vi "3D Major Grid.vi"(5 "Grid Plane Visible":T1, 6 "Inverted?":bool, 7 "Axis":enum16{"X-Axis", "Y-Axis", "Z-Axis"}(ring), 8 "error in (no error)":errorcluster, 9 "Grid Color":u32(colorbox), 10 "Range":cluster{"Max":sgl, "Min":sgl}, 11 "Tick Cluster Array":T2) -> (0 "error out":errorcluster, 3 "Grid Object Out":refnum<vi>)   [LabVIEW 2013]
uses:
  <vilib>/Math Plots/3D Math Plots/3D Plot/3D Plot/Typedef/Tick Array.ctl
  <vilib>/picture/3D Picture Control/Object/Create Object (name).vi
  <vilib>/picture/3D Picture Control/NI_3D Picture Control.lvlib
  <vilib>/Math Plots/3D Math Plots/3D Plot/3D Plot/3D Plot.lvclass
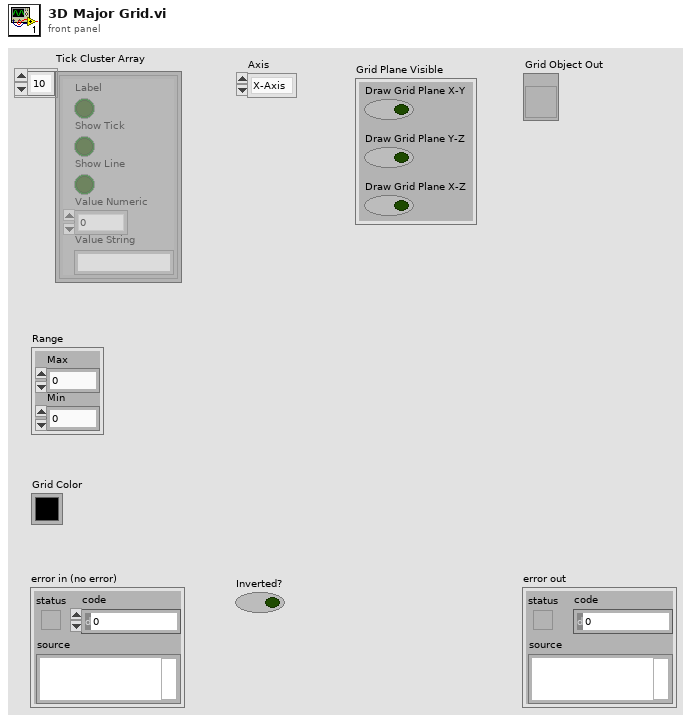
[diagram p1: front panel]
types:
  T1 = cluster{"Draw Grid Plane X-Y":bool, "Draw Grid Plane Y-Z":bool, "Draw Grid Plane X-Z":bool}
  T2 = typedef "3D Plot.lvclass/Tick Array.ctl" = cluster{"Label":bool, "Show Tick":bool, "Show Line":bool, "Value Numeric":sgl, "Value String":string}[]
  T3 = enum16{"Overall", "Per Primitive", "Per Vertex", "Binding Off"}
  T4 = enum16{"Points", "Lines", "Line Strip", "Line Loop", "Triangles", "Triangle Strip", "Triangle Fan", "Quads", "Quad Strip", "Polygon"}
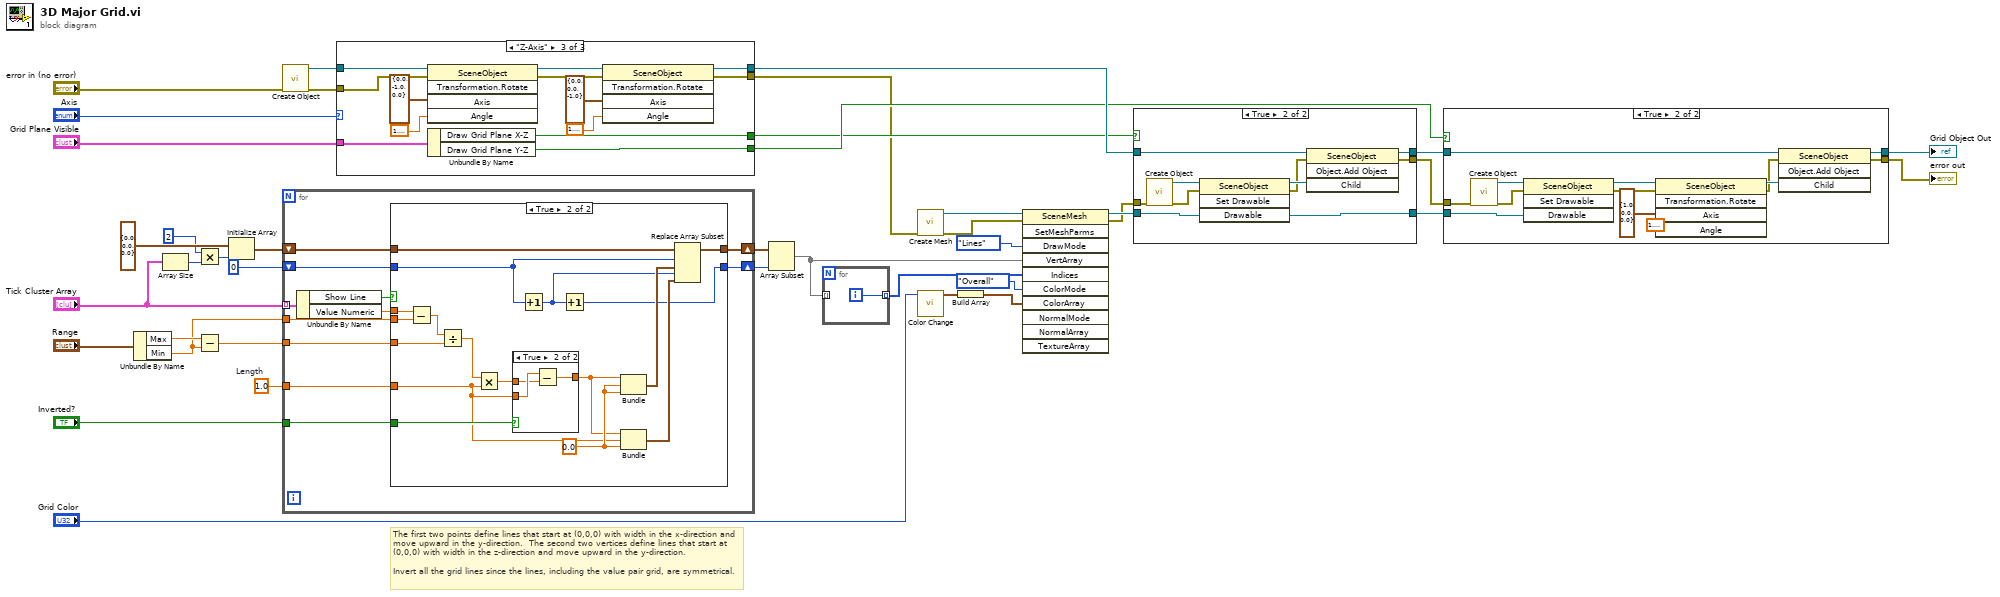
[diagram p0: block diagram]
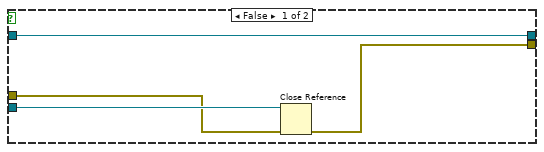
[diagram p2: hidden frame]
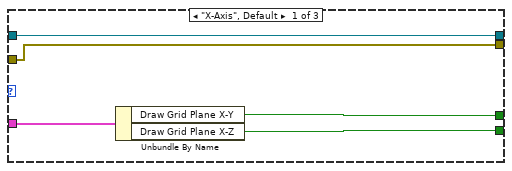
[diagram p3: hidden frame]
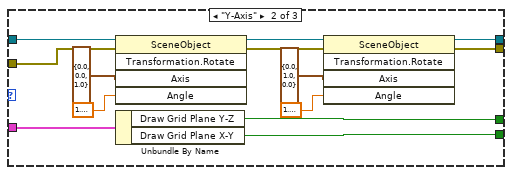
[diagram p4: hidden frame]
diagram:
  w40 = sgl 1.0  # Length
  # "The first two points define lines that start at (0,0,0) with width in the x-direction and move upward in the y-direction.  The second two vertices define lines that start at (0,0,0) with width in the z-direction and move upward in the y-direction.\n\nInvert all the grid lines since the lines, including the value pair grid, are symmetrical."
  n1 = Unbundle By Name("Range") -> ("Max"=w29:sgl, "Min"=w28:sgl)
  n2 = Array Size(array="Tick Cluster Array") -> (size(s)=w6:i32)
  n3 = Multiply(x=2 ("y"), y=w6) -> (x*y=w2:i32)
  n4 = Subtract(x=w29, y=w28) -> (x-y=w30:sgl)
  n5 = Initialize Array(cluster{"X":sgl, "Y":sgl, "Z":sgl} {"X"=0.0, "Y"=0.0, "Z"=0.0} ("3D Point"), w2) -> (w7:cluster{"X":sgl, "Y":sgl, "Z":sgl}[])
  n6 = call-poly <vilib>:"Create Object.vi"("error in (no error)"="error in (no error)") -> ("error out"=w14:errorcluster, "Scene:New Object"=w15:refnum<vi>)  [unwired: 9 in]
  n7 = for {
    tunnel: "Tick Cluster Array" -> [w51] mode=indexing
    tunnel: w28 -> [w49]
    tunnel: w40 -> [w44]
    tunnel: w30 -> [w48]
    shift-right: [w46] -> w9
    shift-left: w7 -> [w47]
    tunnel: "Inverted?" -> [w45]
    shift-right: [w42] -> w3
    shift-left: 0 -> [w43]
    n8 = Unbundle By Name(w51) -> ("Show Line"=w41:bool, "Value Numeric"=w50:sgl)
    n9 = case shown="True" w41 {
      tunnel: w50 -> [_ w70]
      tunnel: w49 -> [_ w69]
      tunnel: w48 -> [_ w67]
      tunnel: w47 -> [w53 w65]
      tunnel: [w53 w64] -> w46
      tunnel: w45 -> [_ w62]
      tunnel: w44 -> [_ w60]
      tunnel: w43 -> [w52 w56]
      tunnel: [w52 w54] -> w42
      frame False {
      }
      frame True {
        w61 = sgl 0.0 ("x*y")
        n10 = Subtract(x=w70, y=w69) -> (x-y=w68:sgl)
        n11 = Divide(x=w68, y=w67) -> (x/y=w66:sgl)
        n12 = Multiply(x=w66, y=w60) -> (x*y=w63:sgl)
        n13 = case shown="True" w62 {
          tunnel: w63 -> [w71 w73]
          tunnel: w60 -> [_ w74]
          tunnel: [w71 w72] -> w59
          frame False {
          }
          frame True {
            n14 = Subtract(x=w74, y=w73) -> (x-y=w72:sgl)
          }
        }
        n15 = Increment(x=w56) -> (x+1=w55:i32)
        n16 = Increment(x=w55) -> (x+1=w54:i32)
        n17 = Bundle(w59, "x*y"=w61, "x*y"=w61) -> (w58:cluster{sgl, "x*y":sgl, "x*y":sgl})  [unwired: 1 out]
        n18 = Bundle(w59, "Length"=w60, "x*y"=w61) -> (w57:cluster{sgl, "Length":sgl, "x*y":sgl})  [unwired: 1 out]
        n19 = Replace Array Subset(array=w65, new element #1=w58, index #1=w56, new element #2=w57, index #2=w55) -> (w64:cluster{"X":sgl, "Y":sgl, "Z":sgl}[])
      }
    }
  }
  n20 = case shown="\"Z-Axis\"" "Axis" {
    tunnel: [w79 w83 w97] -> w16
    tunnel: w15 -> [w79 w86 w99]
    tunnel: [w78 w84 w98] -> w11
    tunnel: w14 -> [w78 w85 w96]
    tunnel: "Grid Plane Visible" -> [w77 w82 w95]
    tunnel: [w76 w81 w94] -> w13
    tunnel: [w75 w80 w93] -> w12
    frame "X-Axis", Default {
      n21 = Unbundle By Name(w77) -> ("Draw Grid Plane X-Y"=w75:bool, "Draw Grid Plane X-Z"=w76:bool)
    }
    frame "Y-Axis" {
      n22 = invoke class="SceneObject" method="Transformation.Rotate"(reference=w86, error in=w85, "Axis"=cluster{"X":sgl, "Y":sgl, "Z":sgl} {"X"=0.0, "Y"=0.0, "Z"=1.0}, "Angle"=1.5707963267948966) -> (reference out=w91:refnum<vi>, error out=w92:errorcluster)  [unwired: 1 in, 3 out]
      n23 = Unbundle By Name(w82) -> ("Draw Grid Plane Y-Z"=w80:bool, "Draw Grid Plane X-Y"=w81:bool)
      n24 = invoke class="SceneObject" method="Transformation.Rotate"(reference=w91, error in=w92, "Axis"=cluster{"X":sgl, "Y":sgl, "Z":sgl} {"X"=0.0, "Y"=1.0, "Z"=0.0}, "Angle"=1.5707963267948966) -> (reference out=w83:refnum<vi>, error out=w84:errorcluster)  [unwired: 1 in, 3 out]
    }
    frame "Z-Axis" {
      n25 = invoke class="SceneObject" method="Transformation.Rotate"(reference=w99, error in=w96, "Axis"=cluster{"X":sgl, "Y":sgl, "Z":sgl} {"X"=0.0, "Y"=-1.0, "Z"=0.0}, "Angle"=1.5707963267948966) -> (reference out=w100:refnum<vi>, error out=w105:errorcluster)  [unwired: 1 in, 3 out]
      n26 = Unbundle By Name(w95) -> ("Draw Grid Plane X-Z"=w93:bool, "Draw Grid Plane Y-Z"=w94:bool)
      n27 = invoke class="SceneObject" method="Transformation.Rotate"(reference=w100, error in=w105, "Axis"=cluster{"X":sgl, "Y":sgl, "Z":sgl} {"X"=0.0, "Y"=0.0, "Z"=-1.0}, "Angle"=1.5707963267948966) -> (reference out=w97:refnum<vi>, error out=w98:errorcluster)  [unwired: 1 in, 3 out]
    }
  }
  n28 = Array Subset(array=w9, length=w3) -> (w4:cluster{"X":sgl, "Y":sgl, "Z":sgl}[])  [unwired: 1 in]
  n29 = for {
    tunnel: w4 -> [_] mode=indexing
    tunnel: [w106] -> w20 mode=indexing
    i -> [w106]
  }
  n30 = call <vilib>:"Create Mesh.vi"("error in (no error)"=w11) -> ("error out"=w27:errorcluster, "New Mesh Refnum"=w22:refnum<vi>)  [unwired: 9 out]
  n31 = call <vilib>:"Color Change.vi"("Color"="Grid Color") -> ("RGBA"=w21:cluster{"R":sgl, "G":sgl, "B":sgl, "A":sgl})  [unwired: 1 in, 9 out]
  n32 = Build Array(w21) -> (w25:cluster{"R":sgl, "G":sgl, "B":sgl, "A":sgl}[])
  n33 = invoke class="SceneMesh" method="SetMeshParms"(reference=w22, error in=w27, "DrawMode"=T4."Lines" ("Draw Mode"), "VertArray"=w4, "Indices"=w20, "ColorMode"=T3."Overall" ("Color Binding Mode"), "ColorArray"=w25) -> (reference out=w26:refnum<vi>, error out=w10:errorcluster)  [unwired: 4 in, 9 out]
  n34 = case shown="True" w12 {
    tunnel: w26 -> [w107 w118]
    tunnel: [w107 w116] -> w17
    tunnel: [w108 w110] -> w19
    tunnel: [w109 w114] -> w18
    tunnel: w16 -> [w109 w113]
    tunnel: w10 -> [w108 w112]
    frame False {
    }
    frame True {
      n35 = call-poly <vilib>:"Create Object.vi"("error in (no error)"=w112) -> ("error out"=w119:errorcluster, "Scene:New Object"=w117:refnum<vi>)  [unwired: 9 in]
      n36 = invoke class="SceneObject" method="Set Drawable"(reference=w117, error in=w119, "Drawable"=w118) -> (reference out=w115:refnum<vi>, error out=w111:errorcluster, "Drawable"=w116:refnum<vi>)  [unwired: 1 in, 1 out]
      n37 = invoke class="SceneObject" method="Object.Add Object"(reference=w113, error in=w111, "Child"=w115) -> (reference out=w114:refnum<vi>, error out=w110:errorcluster)  [unwired: 1 in, 2 out]
    }
  }
  n38 = case shown="True" w13 {
    tunnel: w19 -> [w121 w134]
    tunnel: w18 -> [w123 w133]
    tunnel: [w123 w132] -> w36
    tunnel: [w120 w131] -> w35
    tunnel: w17 -> [w122 w127]
    frame False {
      n39 = Close Reference(reference=w122, error in (no error)=w121) -> (error out=w120:errorcluster)
    }
    frame True {
      n40 = call-poly <vilib>:"Create Object.vi"("error in (no error)"=w134) -> ("error out"=w128:errorcluster, "Scene:New Object"=w129:refnum<vi>)  [unwired: 9 in]
      n41 = invoke class="SceneObject" method="Set Drawable"(reference=w129, error in=w128, "Drawable"=w127) -> (reference out=w126:refnum<vi>, error out=w125:errorcluster)  [unwired: 1 in, 2 out]
      n42 = invoke class="SceneObject" method="Transformation.Rotate"(reference=w126, error in=w125, "Axis"=cluster{"X":sgl, "Y":sgl, "Z":sgl} {"X"=1.0, "Y"=0.0, "Z"=0.0}, "Angle"=sgl 1.5707964) -> (reference out=w130:refnum<vi>, error out=w124:errorcluster)  [unwired: 1 in, 3 out]
      n43 = invoke class="SceneObject" method="Object.Add Object"(reference=w133, error in=w124, "Child"=w130) -> (reference out=w132:refnum<vi>, error out=w131:errorcluster)  [unwired: 1 in, 2 out]
    }
  }
  "Grid Object Out" <- w36
  "error out" <- w35
